vi "Save Default Client Mediator Settings to XML FIles_Core.vi"() -> ()   [LabVIEW 2014]
uses:
  <vilib>/Utility/xml.llb/Write to XML File(string).vi
panel:
  out "error out med":errorcluster
  out "error out cli":errorcluster
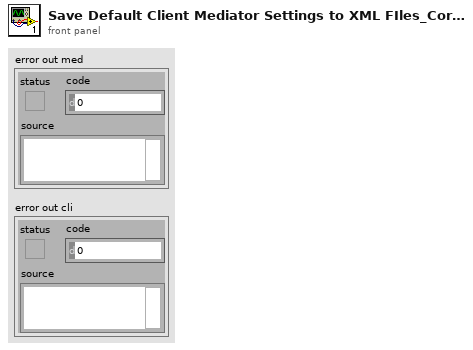
[diagram p1: front panel]
types:
  T1 = typedef "System_Settings_Cluster_Client_Mediator_Core.ctl" = cluster{"Units in the system":T2[], "dBase names by units":string[], "TCP/IP processing units addresses":string[], "TCP/IP server address":string, "dBase User Name_Cli":string, "dBase User Password_Cli":string, "dBase User Name_Med":string, "dBase User Password_Med":string, "Sampling rate [Hz]":dbl, "FTP Server User name, cRIO":string, "FTP Server Password, cRIO":string, "OnScreenKeyboardPopUp":bool, "Number of points to collect":u32, "Main Window has title bar?":bool, "Demo?":bool, "dBase - Limit # of  elements to read":u32, "dBase Backup":cluster{"dBase Backup Base Folder":string, "Remote dBase Backup Configured?":bool}, "System Status":cluster{"System Monitor Refresh Rate (ms)":u32, "System Status Log  File":string, "Max number of elements to read\n":i64}, "Number of points to average for stationary state":i32[], "Number of points to collect for saving waveforms per channel":i32[], "Sources per Unit":T3[], "TCP/IP_client_mediator_communication ports":u16, "TCP/IP processing_units _mediator_communication ports":u16}
  T2 = typedef "Unit_Names_Core.ctl" = enum16{"Not used", "Unit 1", "Unit 2", "Unit 3", "Unit 4", "Unit 5", "Unit 6", "Unit 7", "Unit 8", "Unit 9"}
  T3 = typedef "Data_Sources_Core.ctl" = enum16{"Not Used", "Source 0", "Source 1", "Source 2", "Source 3", "Source 4", "Source 5", "Source 6", "Source 7", "Source 8", "Source 9", "Source 10", "Source 11", "Source 12", "Source 13", "Source 14", "Source 15", "Source 16", "Source 17", "Source 18", "Source 19", "Source 20"}
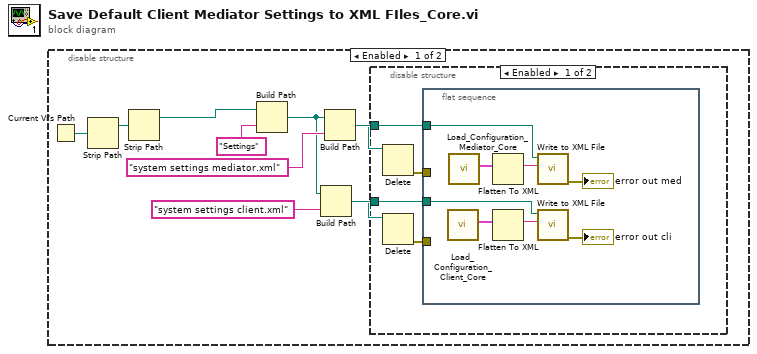
[diagram p0: block diagram]
diagram:
  n1 = disable-structure shown="Enabled" {
    frame Enabled {
      n2 = Current VI's Path() -> (path=w9:path)
      n3 = Strip Path(path=w9) -> (stripped path=w8:path)  [unwired: 1 out]
      n4 = Strip Path(path=w8) -> (stripped path=w1:path)  [unwired: 1 out]
      n5 = Build Path(base path=w1, name or relative path="Settings") -> (appended path=w5:path)
      n6 = Build Path(base path=w5, name or relative path="system settings client.xml") -> (appended path=w2:path)
      n7 = Build Path(base path=w5, name or relative path="system settings mediator.xml") -> (appended path=w3:path)
      n8 = disable-structure shown="Enabled" {
        disable-tunnel: w3 -> [w13 _]
        disable-tunnel: w2 -> [w11 _]
        frame Enabled {
          n9 = Delete(path (use dialog)=w13) -> (error out=w12:errorcluster)  [unwired: 4 in, 2 out]
          n10 = Delete(path (use dialog)=w11) -> (error out=w10:errorcluster)  [unwired: 4 in, 2 out]
          n11 = flat-sequence {
            tunnel: w13 -> [w15]
            tunnel: w11 -> [w14]
            tunnel: w12 -> [_]
            tunnel: w10 -> [_]
            frame #0 {
              n12 = call "Load_Configuration_Client_Core.vi"() -> ("System_settings OUT"=w19:T1)  [unwired: 11 out]
              n13 = call "Load_Configuration_Mediator_Core.vi"() -> ("System_settings OUT"=w18:T1)  [unwired: 11 in]
              n14 = Flatten To XML(anything=w18) -> (xml string=w20:string)
              n15 = Flatten To XML(anything=w19) -> (xml string=w21:string)
              n16 = call-poly <vilib>:"Write to XML File.vi"("XML Input"=w20, "XML File Path"=w15) -> ("error out"=→"error out med":errorcluster)  [unwired: 7 in, 2 out]
              n17 = call-poly <vilib>:"Write to XML File.vi"("XML Input"=w21, "XML File Path"=w14) -> ("error out"=→"error out cli":errorcluster)  [unwired: 7 in, 2 out]
            }
          }
        }
        frame Disabled {
        }
      }
    }
    frame Disabled {
    }
  }
